vi "alternate.vi"(0 "iteration":i32) -> (4 "message":string)   [LabVIEW 2026]
doc: "Returns \"hello world\" on even iterations and an empty string on odd ones, so wiring it to a loop's iteration terminal makes text appear and vanish on alternating cycles.\n\nMeant to be dropped inside the Timed Loop of tl.vi: wire the loop's iteration terminal (i) to iteration, and message to a string indicator."
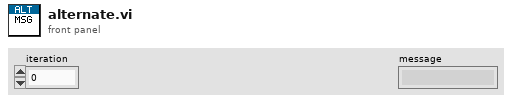
[diagram p1: front panel]
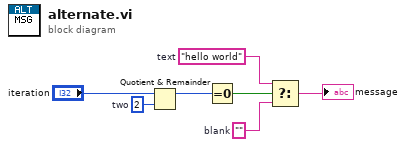
[diagram p0: block diagram]
diagram:
  w2 = ""  # blank
  w4 = "hello world"  # text
  w6 = 2  # two
  n1 = Quotient & Remainder(x="iteration", y=w6) -> (x-y*floor(x/y)=w5:i32)  [unwired: 1 out]
  n2 = Equal To 0?(x=w5) -> (x = 0?=w3:bool)
  n3 = Select(t=w4, s=w3, f=w2) -> (s? t:f=→"message":string)
